vi "Load User.vi"(7 "User Name 2":string, 8 "error in (no error)":errorcluster, 11 "Programing Logic in":refnum<class "Programing Logic.lvclass">) -> (0 "error out":errorcluster, 3 "Programing Logic out":refnum<class "Programing Logic.lvclass">)   [LabVIEW 2014, in "Programing Logic.lvclass"]
uses:
  Programming Logic/Programing Logic.lvclass
  Programming Logic/Programing Logic.lvclass/Programing Logic.ctl
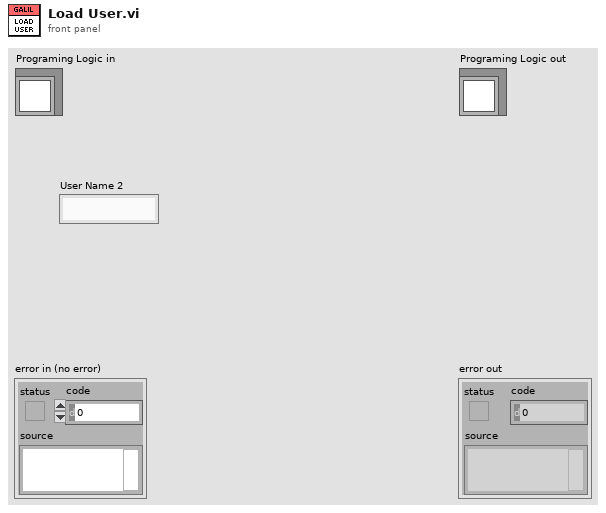
[diagram p1: front panel]
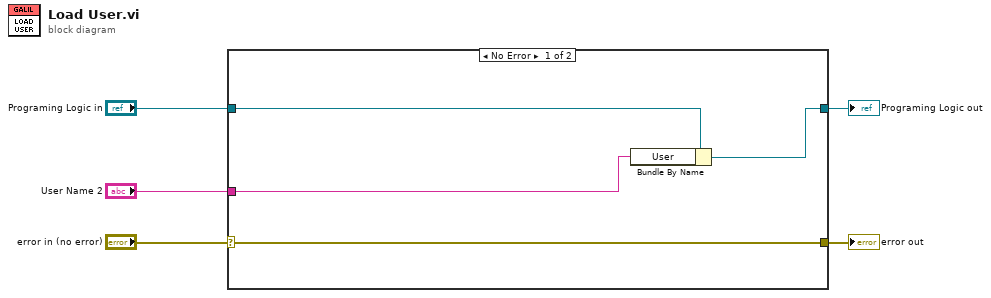
[diagram p0: block diagram]
diagram:
  n1 = case shown="No Error" "error in (no error)" {
    selector: "error in (no error)" -> [w9 w11]
    tunnel: [w9 w11] -> w4
    tunnel: [w7 w10] -> w2
    tunnel: "Programing Logic in" -> [w8 w10]
    tunnel: "User Name 2" -> [w6 _]
    frame No Error {
      n2 = Bundle By Name(cluster=w8, "User"=w6) -> (w7:refnum<class "Programing Logic.lvclass">)
    }
    frame Error {
    }
  }
  "error out" <- w4
  "Programing Logic out" <- w2
